vi "CONEX Module.vi"(0 "Device Cfg [In]":variant, 1 "Actions":T2(ring)=enum."Stop", 5 "Connected [In]":bool, 11 "Error In":errorcluster, 12 "Stage Limits":cluster{"Lower Limit":dbl, "Upper Limit":dbl}) -> (4 "Device Cfg [Out]":variant, 6 "Connected [Out]":bool, 10 "Current position":dbl, 14 "Timout Error":bool, 15 "Error Out":errorcluster)   [LabVIEW 2014]
uses:
  General/Controls/TableStageModels.ctl
panel:
  in  "Stage Types":T1
  in  "Abs Pos.":dbl
  in  "Step Size":dbl
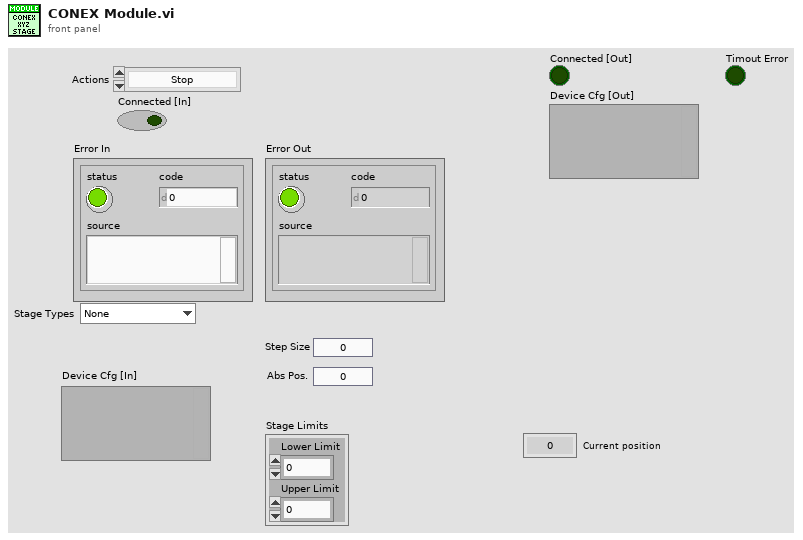
[diagram p1: front panel]
types:
  T1 = typedef "TableStageModels.ctl" = enum16{"None", "CONEX-CC"}
  T2 = enum16{"Unknown", "Init", "Connect", "Step", "Move", "Stop", "Get Position", "Set Limits", "Disconnect"}
  T3 = cluster{"VISA resource name":refnum<visa-resource-name>, "Device name":string, "Controller address":i32, "error":errorcluster}
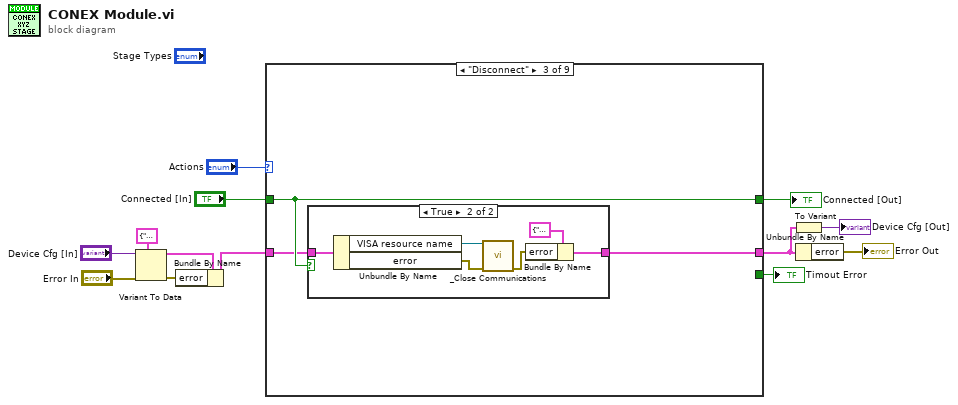
[diagram p0: block diagram]
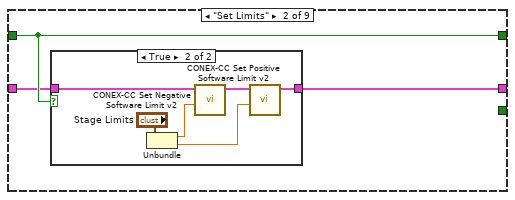
[diagram p3: hidden frame]
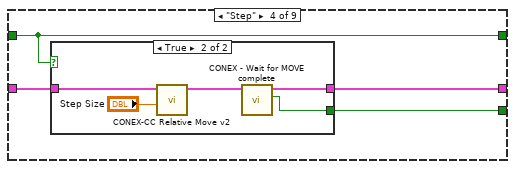
[diagram p6: hidden frame]
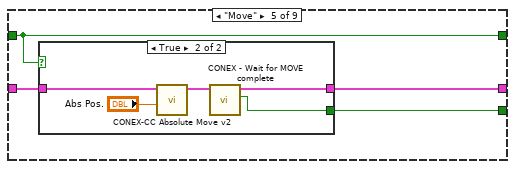
[diagram p8: hidden frame]
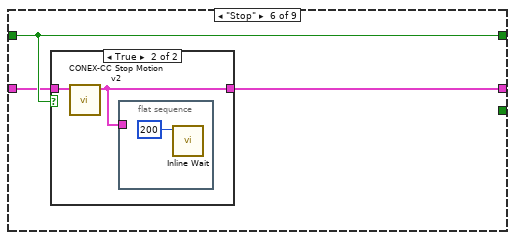
[diagram p10: hidden frame]
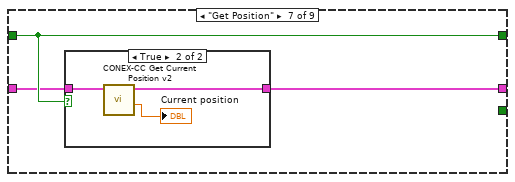
[diagram p12: hidden frame]
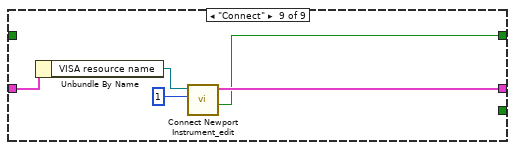
[diagram p15: hidden frame]
diagram:
  n1 = Variant To Data(error in="Error In", type=T3 {"VISA resource name"="", "Device name"="", "Controller address"=0, "error"={"status"=FALSE, "code"=0, "source"=""}} ("Device Connection Cluster [In]"), Variant="Device Cfg [In]") -> (data=w4:T3, error out=w3:errorcluster)
  n2 = Bundle By Name(cluster=w4, "error"=w3) -> (w10:T3)
  n3 = case shown="\"Disconnect\"" "Actions" {
    tunnel: [_ w14 w24 w35 w45 w54 w61 w69 w73] -> w2
    tunnel: w10 -> [_ w15 w25 w36 w46 w55 w62 w69 w71]
    tunnel: [_ w16 w26 w37 w47 w56 w63 w68 w72] -> w11
    tunnel: "Connected [In]" -> [_ w16 w26 w37 w47 w56 w63 w68 _]
    tunnel: [_ _ _ w34 w44 _ _ _ _] -> w8
    frame "Init" {
    }
    frame "Set Limits" {
      n4 = case shown="True" w16 {
        tunnel: w15 -> [w17 w22]
        tunnel: [w17 w21] -> w14
        frame False {
        }
        frame True {
          n5 = Unbundle("Stage Limits") -> ("Lower Limit"=w19:dbl, "Upper Limit"=w18:dbl)
          n6 = call "CONEX-CC Set Negative Software Limit v2.vi"("Negative limit (left)"=w19, "Connection Cluster in"=w22) -> ("Connection Cluster out"=w23:T3)  [unwired: 9 in]
          n7 = call "CONEX-CC Set Positive Software Limit v2.vi"("Positive limit (right)"=w18, "Connection Cluster in"=w23) -> ("Connection Cluster out"=w21:T3)  [unwired: 9 in]
        }
      }
    }
    frame "Disconnect" {
      n8 = case shown="True" w26 {
        tunnel: w25 -> [w27 w33]
        tunnel: [w27 w28] -> w24
        frame False {
        }
        frame True {
          n9 = Unbundle By Name(w33) -> ("VISA resource name"=w32:refnum<visa-resource-name>, "error"=w31:errorcluster)
          n10 = call "_Close Communications.vi"("Instrument Channel"=w32, "error in (no error)"=w31) -> ("error out"=w29:errorcluster)  [unwired: 13 in]
          n11 = Bundle By Name(cluster=T3 {"VISA resource name"="", "Device name"="", "Controller address"=0, "error"={"status"=FALSE, "code"=0, "source"=""}} ("Device Connection Cluster"), "error"=w29) -> (w28:T3)
        }
      }
    }
    frame "Step" {
      n12 = case shown="True" w37 {
        tunnel: w36 -> [w38 w42]
        tunnel: [w38 w40] -> w35
        tunnel: [_ w39] -> w34
        frame False {
        }
        frame True {
          n13 = call "CONEX-CC Relative Move v2.vi"("Relative displacement"="Step Size", "Connection Cluster in"=w42) -> ("Connection Cluster out"=w41:T3)  [unwired: 9 in]
          n14 = call "CONEX - Wait for MOVE complete.vi"("Connection Cluster in"=w41) -> ("Timout Error"=w39:bool, "Connection Cluster out"=w40:T3)  [unwired: 9 in]
        }
      }
    }
    frame "Move" {
      n15 = case shown="True" w47 {
        tunnel: w46 -> [w48 w52]
        tunnel: [w48 w50] -> w45
        tunnel: [_ w49] -> w44
        frame False {
        }
        frame True {
          n16 = call "CONEX-CC Absolute Move v2.vi"("Target position"="Abs Pos.", "Connection Cluster in"=w52) -> ("Connection Cluster out"=w51:T3)  [unwired: 7 in]
          n17 = call "CONEX - Wait for MOVE complete.vi"("Connection Cluster in"=w51) -> ("Timout Error"=w49:bool, "Connection Cluster out"=w50:T3)  [unwired: 9 in]
        }
      }
    }
    frame "Stop" {
      n18 = case shown="True" w56 {
        tunnel: w55 -> [w57 w59]
        tunnel: [w57 w58] -> w54
        frame False {
        }
        frame True {
          n19 = call "CONEX-CC Stop Motion v2.vi"("Connection Cluster in"=w59) -> ("Connection Cluster out"=w58:T3)  [unwired: 10 in]
          n20 = flat-sequence {
            tunnel: w58 -> [_]
            frame #0 {
              n21 = call "Inline Wait.vi"("milliseconds to wait"=u32 200) -> ()  [unwired: 10 in, 1 out]
            }
          }
        }
      }
    }
    frame "Get Position" {
      n22 = case shown="True" w63 {
        tunnel: w62 -> [w64 w67]
        tunnel: [w64 w66] -> w61
        frame False {
        }
        frame True {
          n23 = call "CONEX-CC Get Current Position v2.vi"("Connection Cluster in"=w67) -> ("Current position"=→"Current position":dbl, "Connection Cluster out"=w66:T3)  [unwired: 8 in, 1 out]
        }
      }
    }
    frame "Unknown", Default {
    }
    frame "Connect" {
      n24 = Unbundle By Name(w71) -> ("VISA resource name"=w70:refnum<visa-resource-name>)
      n25 = call "Connect Newport Instrument_edit.vi"("Numeric"=i8 1, "String"=w70) -> ("Connected"=w72:bool, "Device Connection Cluster"=w73:T3)  [unwired: 5 in, 3 out]
    }
  }
  "Connected [Out]" <- w11
  "Timout Error" <- w8
  n26 = To Variant(anything=w2) -> (Variant=→"Device Cfg [Out]":variant)
  n27 = Unbundle By Name(w2) -> ("error"=→"Error Out":errorcluster)
